vi "Lab2.vi"() -> ()   [LabVIEW 2010]
uses:
  <vilib>/measure/maspectr.llb/FFT Spectrum (Mag-Phase) for 1 Chan.vi
  <vilib>/measure/NI_MABase.lvlib
  <vilib>/measure/NI_MAPro.lvlib
panel:
  out "Filtered":dynamicdata(graph)
  out "FFT":cluster{"f0":dbl, "df":dbl, "magnitude":dbl[]}(graph)
  in  "stop":bool
  out "Waveform Graph":waveform(dbl)(graph)
  in  "standard deviation":dbl(slide)=1.0 scale=0.0..2.0
  in  "frequency":dbl(slide)=10.0 scale=0.0..10.0
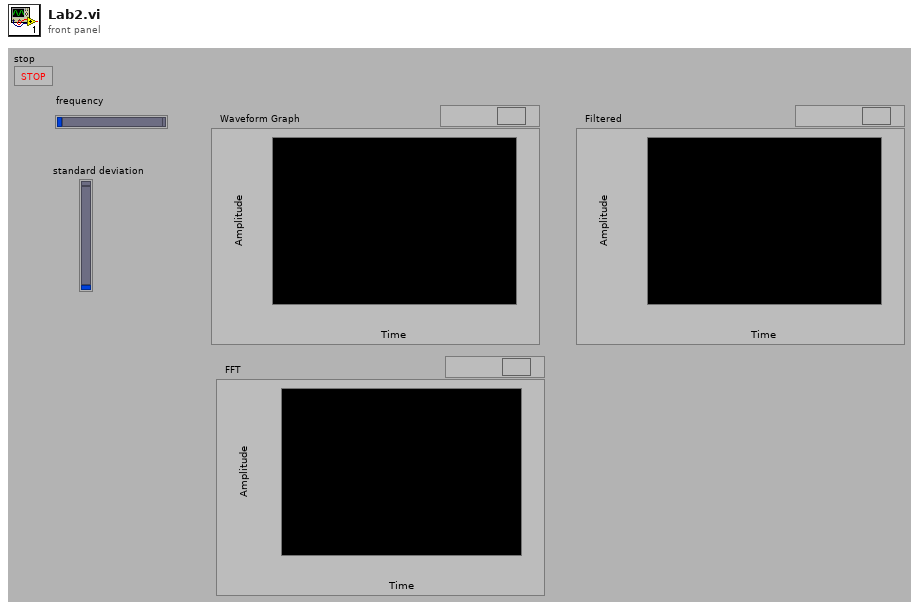
[diagram p1: front panel]
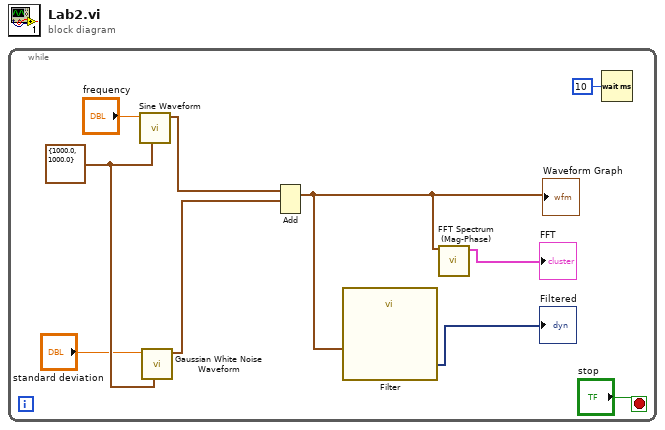
[diagram p0: block diagram]
diagram:
  n1 = while {
    stop <- "stop" stop-if-true
    w9 = cluster{"Fs":dbl, "#s":dbl} {"Fs"=1000.0, "#s"=1000.0} ("sampling info")
    n2 = call <vilib>:"Sine Waveform.vi"("sampling info"=w9, "frequency"="frequency") -> ("signal out"=w7:waveform(dbl))  [unwired: 8 in, 1 out]
    n3 = call <vilib>:"Gaussian White Noise Waveform.vi"("sampling info"=w9, "standard deviation"="standard deviation") -> ("signal out"=w6:waveform(dbl))  [unwired: 8 in, 1 out]
    n4 = Add(1:w6, 2:w7) -> (0:w2:waveform(dbl))  [unwired: 1 in, 1 out]
    "Waveform Graph" <- w2
    n5 = call "Filter"("Signal"=w2) -> ("Filtered Signal"=→"Filtered":dynamicdata)  [unwired: 9 in, 1 out]
    n6 = call-poly <vilib>:"FFT Spectrum (Mag-Phase).vi"("time signal"=w2) -> ("magnitude"=→"FFT":cluster{"f0":dbl, "df":dbl, "magnitude":dbl[]})  [unwired: 6 in, 4 out]
    n7 = Wait (ms)(milliseconds to wait=u32 10) -> ()  [unwired: 1 out]
  }
